vi "VI Server Launcher23.vi"() -> ()   [LabVIEW 2021]
uses:
  363d3bde-6874-4068-849e-62e045d4c070.vi
  <vilib>/Comparison/Less/Less Functor/Less Functor.lvclass
  <vilib>/Utility/LVLibp/NI_PackedLibraryUtility.lvlib
panel:
  out "error out":errorcluster
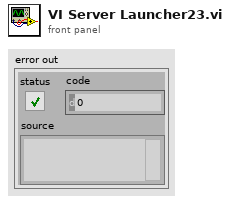
[diagram p1: front panel]
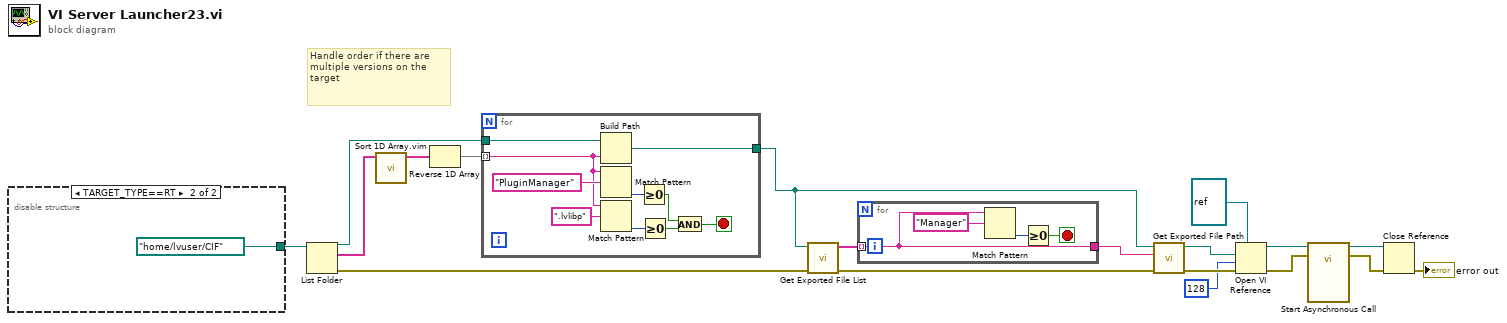
[diagram p0: block diagram]
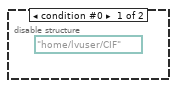
[diagram p2: hidden frame]
diagram:
  # "Handle order if there are multiple versions on the target"
  n1 = disable-structure shown="TARGET_TYPE==RT" {
    disable-tunnel: [_ path "/home/lvuser/CIF" ("packed library path")] -> w19
    frame condition #0 {
      (unwired) path "/home/lvuser/CIF" ("packed library path")
    }
    frame condition #1 (active) {
    }
  }
  n2 = List Folder(path=w19) -> (path out=w17:path, filenames=w14:string[], error out=w18:errorcluster)  [unwired: 3 in, 1 out]
  n3 = call "Sort 1D Array.vim"("unsorted array"=w14) -> ("sorted array"=w13:string[])  [unwired: 10 in]
  n4 = Reverse 1D Array(array=w13) -> (reversed array=w12:string[])
  n5 = for {
    tunnel: w12 -> [w26] mode=indexing
    tunnel: [w27] -> w15
    tunnel: w17 -> [w28]
    stop <- w21 stop-if-true
    n6 = Build Path(base path=w28, name or relative path=w26) -> (appended path=w27:path)
    n7 = Match Pattern(string=w26, regular expression="PluginManager") -> (offset past match=w30:i32)  [unwired: 1 in, 3 out]
    n8 = Match Pattern(string=w26, regular expression=".lvlibp") -> (offset past match=w24:i32)  [unwired: 1 in, 3 out]
    n9 = Greater Or Equal To 0?(x=w30) -> (x >= 0?=w22:bool)
    n10 = Greater Or Equal To 0?(x=w24) -> (x >= 0?=w23:bool)
    n11 = And(x=w22, y=w23) -> (x .and. y?=w21:bool)
  }
  n12 = call <vilib>:"Get Exported File List.vi"("error in (no error)"=w18, "packed library path"=w15) -> ("error out"=w10:errorcluster, "qualified names"=w11:string[])  [unwired: 7 in, 1 out]
  n13 = for {
    tunnel: w11 -> [w31] mode=indexing
    tunnel: [w31] -> w1
    stop <- w33 stop-if-true
    n14 = Match Pattern(string=w31, regular expression="Manager") -> (offset past match=w34:i32)  [unwired: 1 in, 3 out]
    n15 = Greater Or Equal To 0?(x=w34) -> (x >= 0?=w33:bool)
  }
  n16 = call <vilib>:"Get Exported File Path.vi"("error in (no error)"=w10, "qualified name"=w1, "packed library path"=w15) -> ("error out"=w8:errorcluster, "path"=w9:path)  [unwired: 7 in]
  n17 = Open VI Reference(type specifier VI Refnum (for type only)=refnum<vi> refnum, vi path=w9, options=128, error in (no error)=w8) -> (vi reference=w5:refnum<vi>, error out=w4:errorcluster)  [unwired: 2 in]
  n18 = call-by-ref "Start Asynchronous Call"(reference=w5, error in=w4) -> (reference out=w3:refnum<vi>, error out=w2:errorcluster)  [unwired: 12 in]
  n19 = Close Reference(reference=w3, error in (no error)=w2) -> (error out=→"error out":errorcluster)
